vi "Math-Interp1 (1D).vi"(0 "X":dbl[](array[numeric]), 5 "Y":dbl[](array[numeric]), 7 "U":dbl[](array[numeric]), 11 "Default (NaN)":dbl=nan) -> (8 "V":dbl[](array[numeric]))   [LabVIEW 2020]
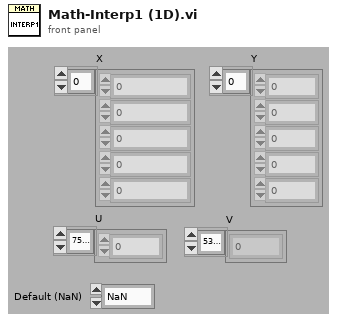
[diagram p1: front panel]
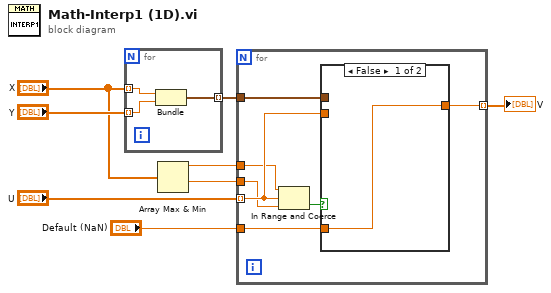
[diagram p0: block diagram]
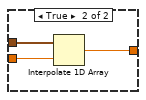
[diagram p2: hidden frame]
diagram:
  n1 = for {
    tunnel: "X" -> [w11] mode=indexing
    tunnel: "Y" -> [w10] mode=indexing
    tunnel: [w9] -> w7 mode=indexing
    n2 = Bundle("Numeric"=w11, "Numeric"=w10) -> (w9:cluster{"Numeric":dbl, "Numeric":dbl})  [unwired: 1 in]
  }
  n3 = Array Max & Min(array="X") -> (max value=w3:dbl, min value=w2:dbl)  [unwired: 2 out]
  n4 = for {
    tunnel: w7 -> [w18]
    tunnel: [w17] -> w5 mode=indexing
    tunnel: "U" -> [w16] mode=indexing
    tunnel: w3 -> [w14]
    tunnel: w2 -> [w15]
    tunnel: "Default (NaN)" -> [w12]
    n5 = In Range and Coerce(upper limit=w14, x=w16, lower limit=w15) -> (In Range?=w13:bool)  [unwired: 1 out]
    n6 = case shown="False" w13 {
      tunnel: w18 -> [_ w22]
      tunnel: [w19 w21] -> w17
      tunnel: w16 -> [_ w20]
      tunnel: w12 -> [w19 _]
      frame False {
      }
      frame True {
        n7 = Interpolate 1D Array(1:w20, 2:w22) -> (0:w21:dbl)
      }
    }
  }
  "V" <- w5
